vi "Filter Item Low Level.vi"(6 "Case Sensitive?":bool, 7 "Filter Type":T1, 8 "error in (no error)":errorcluster, 10 "Filter Value":string, 11 "Item Value":string) -> (0 "error out":errorcluster, 3 "Include?":bool)   [LabVIEW 2020, in "VI Properties Editor.lvlib"]
doc: "Checks whether <B>Item Value</B> will be included in a filter defined by the other inputs."
uses:
  VI Properties Editor.lvlib
  CTLs/Filter Type.ctl
  <vilib>/regexp/Match Regular Expression.xnode
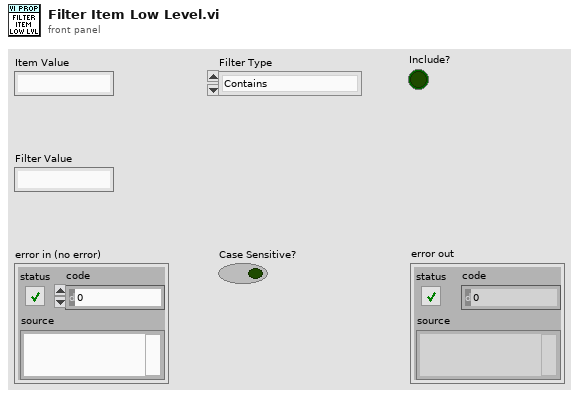
[diagram p1: front panel]
types:
  T1 = typedef "VI Properties Editor.lvlib/Filter Type.ctl" = enum16{"Contains", "Equals", "Starts with", "Ends with", "Is empty", "Does not contain", "Does not equal", "Is not empty"}
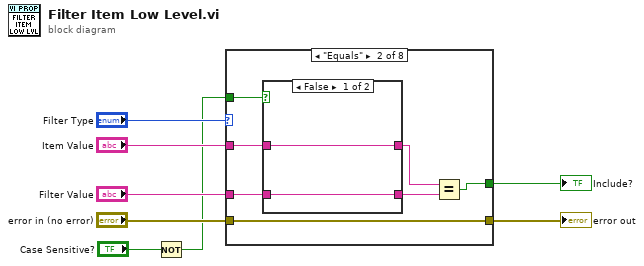
[diagram p0: block diagram]
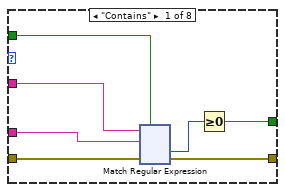
[diagram p2: hidden frame]
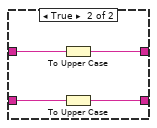
[diagram p3: hidden frame]
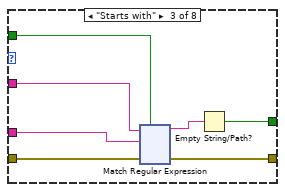
[diagram p4: hidden frame]
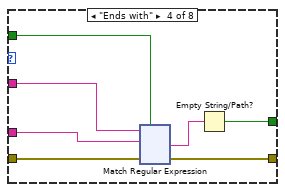
[diagram p5: hidden frame]
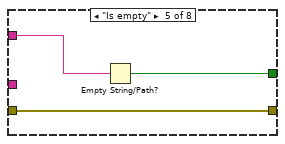
[diagram p6: hidden frame]
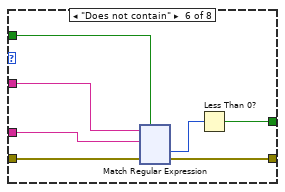
[diagram p7: hidden frame]
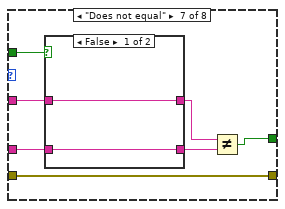
[diagram p8: hidden frame]
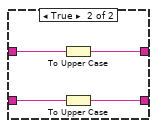
[diagram p9: hidden frame]
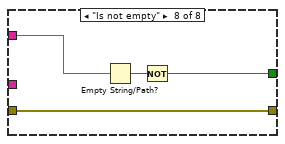
[diagram p10: hidden frame]
diagram:
  n1 = Not(x="Case Sensitive?") -> (.not. x?=w1:bool)
  n2 = case shown="\"Equals\"" "Filter Type" {
    tunnel: "Filter Value" -> [w14 w135 w150 w274 _ w402 w524 _]
    tunnel: "Item Value" -> [w15 w136 w152 w276 w396 w403 w523 w537]
    tunnel: [w12 w139 w151 w275 w395 w400 w527 w534] -> w4
    tunnel: "error in (no error)" -> [w11 w138 w148 w272 w394 w399 w526 w535]
    tunnel: [w10 w138 w147 w271 w394 w398 w526 w535] -> w5
    tunnel: w1 -> [w9 w137 w146 w270 _ w397 w525 _]
    frame "Contains" {
      n3 = xnode "Match Regular Expression"("input string"=w15, "regular expression"=w14, "error in"=w11, "ignore case? (F)"=w9) -> ("offset past match"=w13:i32, "error out"=w10:errorcluster)  [unwired: 2 in, 3 out]
      n4 = Greater Or Equal To 0?(x=w13) -> (x >= 0?=w12:bool)
    }
    frame "Equals" {
      n5 = case shown="False" w137 {
        tunnel: w135 -> [w140 w144]
        tunnel: w136 -> [w141 w145]
        tunnel: [w141 w143] -> w133
        tunnel: [w140 w142] -> w134
        frame False {
        }
        frame True {
          n6 = To Upper Case(1:w145) -> (0:w143:string)
          n7 = To Upper Case(1:w144) -> (0:w142:string)
        }
      }
      n8 = Equal?(x=w133, y=w134) -> (x = y?=w139:bool)
    }
    frame "Starts with" {
      n9 = xnode "Match Regular Expression"("input string"=w152, "regular expression"=w150, "error in"=w148, "ignore case? (F)"=w146) -> ("before match"=w149:string, "error out"=w147:errorcluster)  [unwired: 2 in, 3 out]
      n10 = Empty String/Path?(string/path=w149) -> (empty?=w151:bool)
    }
    frame "Ends with" {
      n11 = xnode "Match Regular Expression"("input string"=w276, "regular expression"=w274, "error in"=w272, "ignore case? (F)"=w270) -> ("after match"=w273:string, "error out"=w271:errorcluster)  [unwired: 2 in, 3 out]
      n12 = Empty String/Path?(string/path=w273) -> (empty?=w275:bool)
    }
    frame "Is empty" {
      n13 = Empty String/Path?(string/path=w396) -> (empty?=w395:bool)
    }
    frame "Does not contain" {
      n14 = xnode "Match Regular Expression"("input string"=w403, "regular expression"=w402, "error in"=w399, "ignore case? (F)"=w397) -> ("offset past match"=w401:i32, "error out"=w398:errorcluster)  [unwired: 2 in, 3 out]
      n15 = Less Than 0?(x=w401) -> (x < 0?=w400:bool)
    }
    frame "Does not equal" {
      n16 = case shown="False" w525 {
        tunnel: w524 -> [w528 w532]
        tunnel: w523 -> [w529 w533]
        tunnel: [w529 w531] -> w522
        tunnel: [w528 w530] -> w521
        frame False {
        }
        frame True {
          n17 = To Upper Case(1:w533) -> (0:w531:string)
          n18 = To Upper Case(1:w532) -> (0:w530:string)
        }
      }
      n19 = Not Equal?(x=w522, y=w521) -> (x != y?=w527:bool)
    }
    frame "Is not empty" {
      n20 = Empty String/Path?(string/path=w537) -> (empty?=w536:bool)
      n21 = Not(x=w536) -> (.not. x?=w534:bool)
    }
  }
  "error out" <- w5
  "Include?" <- w4
